vi "disconnect.vi"(8 "error in":errorcluster, 11 "Nominal Client":refnum<class "Nominal Client.lvclass">) -> (0 "error out":errorcluster)   [LabVIEW 2024, in "nominal labview client.lvlib"]
uses:
  nominal labview client.lvlib
  <vilib>/Nominal/Nominal IO Client/Nominal Client/Nominal Client.lvclass
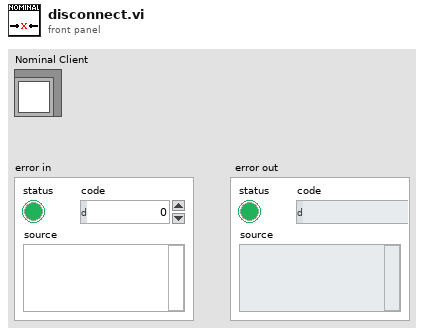
[diagram p1: front panel]
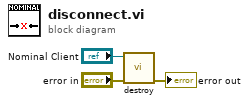
[diagram p0: block diagram]
diagram:
  n1 = call <vilib>:"destroy.vi"("error in"="error in", "Nominal Client"="Nominal Client") -> ("error out"=→"error out":errorcluster)  [unwired: 9 in]
